vi "testing.vi"() -> ()   [LabVIEW 2016]
uses:
  <userlib>/Fluigent/Fluigent MFCS/FluigentMFCS_Full.llb/MFCS_EZ Detect.vi
  <userlib>/Fluigent/Fluigent MFCS/FluigentMFCS_Full.llb/MFCS_EZ Initialization.vi
  <userlib>/Fluigent/Fluigent MFCS/FluigentMFCS_Full.llb/MFCS_EZ Set Channel EV.vi
  <userlib>/Fluigent/Fluigent MFCS/FluigentMFCS_Full.llb/MFCS_EZ Close.vi
panel:
  in  "milliseconds to wait":u32
  out "Waveform Chart 2":dbl(graph)
  out "Waveform Chart":dbl(graph)
  out "All Channels Pressure":dbl[](array[numeric])
  out "error out 2":errorcluster
  out "x-y 2":dbl
  in  "stop 2":bool
  out "error out":errorcluster
  in  "stop":bool
  out "x-y":dbl
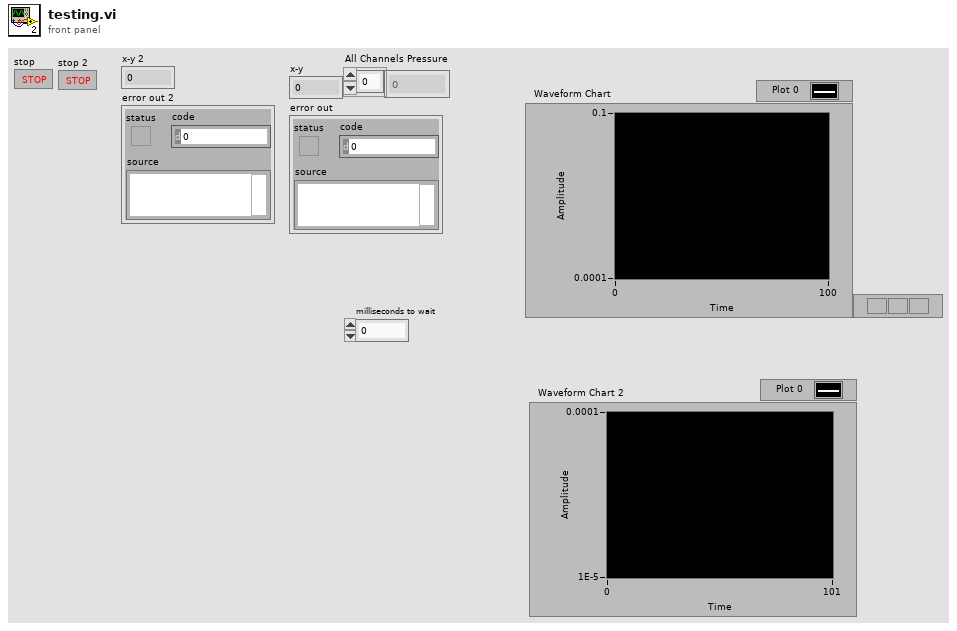
[diagram p1: front panel]
types:
  T1 = typedef "_EZmfcsSN.ctl" = u16
  T2 = typedef "_EZmfcsRefNum.ctl" = refnum<k1>
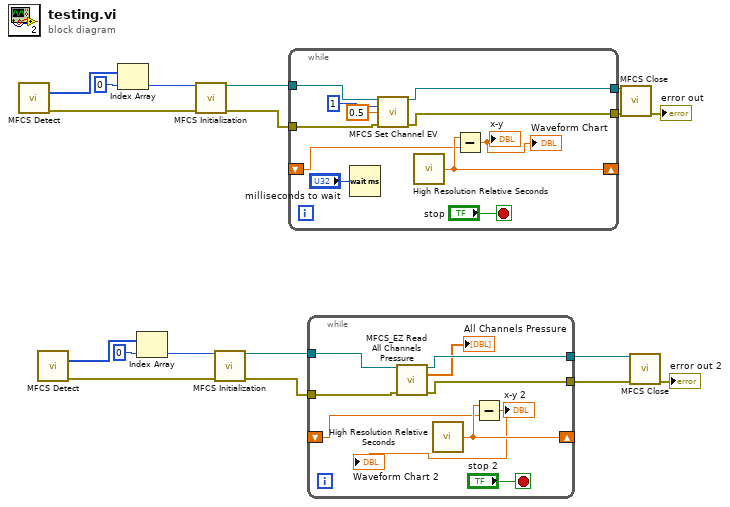
[diagram p0: block diagram]
diagram:
  n1 = call-poly <userlib>:"MFCS Detect.vi"() -> ("[SN MFCS_EZ]"=w18:T1[], "error out"=w15:errorcluster)  [unwired: 14 in]
  n2 = call-poly <userlib>:"MFCS Detect.vi"() -> ("[SN MFCS_EZ]"=w9:T1[], "error out"=w6:errorcluster)  [unwired: 14 in]
  n3 = Index Array(array=w18, index=0) -> (element=w17:T1)
  n4 = Index Array(array=w9, index=0) -> (element=w8:T1)
  n5 = call-poly <userlib>:"MFCS Initialization.vi"("SN MFCS_EZ"=w17, "error in (no error)"=w15) -> ("MFCS_EZ"=w14:T2, "error out"=w12:errorcluster)  [unwired: 11 in, 1 out]
  n6 = call-poly <userlib>:"MFCS Initialization.vi"("SN MFCS_EZ"=w8, "error in (no error)"=w6) -> ("MFCS_EZ"=w5:T2, "error out"=w3:errorcluster)  [unwired: 11 in, 1 out]
  n7 = while {
    tunnel: w14 -> [w28]
    shift-right: [w26] -> _
    shift-left: _ -> [w25]
    tunnel: [w23] -> w13
    tunnel: w12 -> [w22]
    tunnel: [w21] -> w11
    stop <- "stop" stop-if-true
    n8 = Wait (ms)(milliseconds to wait="milliseconds to wait") -> ()  [unwired: 1 out]
    n9 = call-poly <userlib>:"MFCS Set Channel EV.vi"("MFCS_EZ"=w28, "Channel Number (0=All)"=u8 1, "% EV"=sgl 0.5, "error in (no error)"=w22) -> ("MFCS_EZ out"=w23:T2, "error out"=w21:errorcluster)  [unwired: 10 in]
    n10 = call <vilib>:"High Resolution Relative Seconds.vi"() -> ("relative seconds"=w26:dbl)
    n11 = Subtract(x=w26, y=w25) -> (x-y=→"x-y" →"Waveform Chart":dbl)
  }
  n12 = while {
    tunnel: w5 -> [w38]
    shift-right: [w37] -> _
    shift-left: _ -> [w36]
    tunnel: [w34] -> w4
    tunnel: w3 -> [w33]
    tunnel: [w32] -> w2
    stop <- "stop 2" stop-if-true
    n13 = call <userlib>:"MFCS_EZ Read All Channels Pressure.vi"("MFCS_EZ"=w38, "error in (no error)"=w33) -> ("MFCS_EZ out"=w34:T2, "All Channels Pressure"=→"All Channels Pressure":dbl[], "error out"=w32:errorcluster)  [unwired: 11 in]
    n14 = call <vilib>:"High Resolution Relative Seconds.vi"() -> ("relative seconds"=w37:dbl)
    n15 = Subtract(x=w37, y=w36) -> (x-y=→"x-y 2" →"Waveform Chart 2":dbl)
  }
  n16 = call-poly <userlib>:"MFCS Close.vi"("MFCS_EZ"=w13, "error in (no error)"=w11) -> ("error out"=→"error out":errorcluster)  [unwired: 13 in]
  n17 = call-poly <userlib>:"MFCS Close.vi"("MFCS_EZ"=w4, "error in (no error)"=w2) -> ("error out"=→"error out 2":errorcluster)  [unwired: 13 in]
